vi "Tag Based Metadata Interface.vi"(0 "Save Path":path, 7 "Input Tags Path":path) -> ()   [LabVIEW 2020]
uses:
  <vilib>/Utility/miscctls.llb/LVPointTypeDef.ctl
  <vilib>/Utility/file.llb/Read Delimited Spreadsheet (string).vi
panel:
  in  "Clear All Tags":bool
  in  "Group Name Input":string
  in  "Clear Tags":bool
  in  "Remove Group":bool
  in  "Add Group":bool
  in  "Notes":string
  in  "Tag Group 6":bool
  in  "Tag Group 5":bool
  in  "Tag Group 4":bool
  in  "Tag Group 3":bool
  in  "Tag Group 2":bool
  in  "Tag Group 1":bool
  in  "Tag Group 0":bool
  in  "Metadata Tags":string[][](array[string])
  in  "Cancel":bool
  in  "Save":bool
  in  "Update Preset":bool
  in  "Save Preset":bool
  in  "Preset":u16(ring) items=["None", "Apple", "Bean", "My Test", "Test 01", "Test 02", "Test Two", "Zoo"]
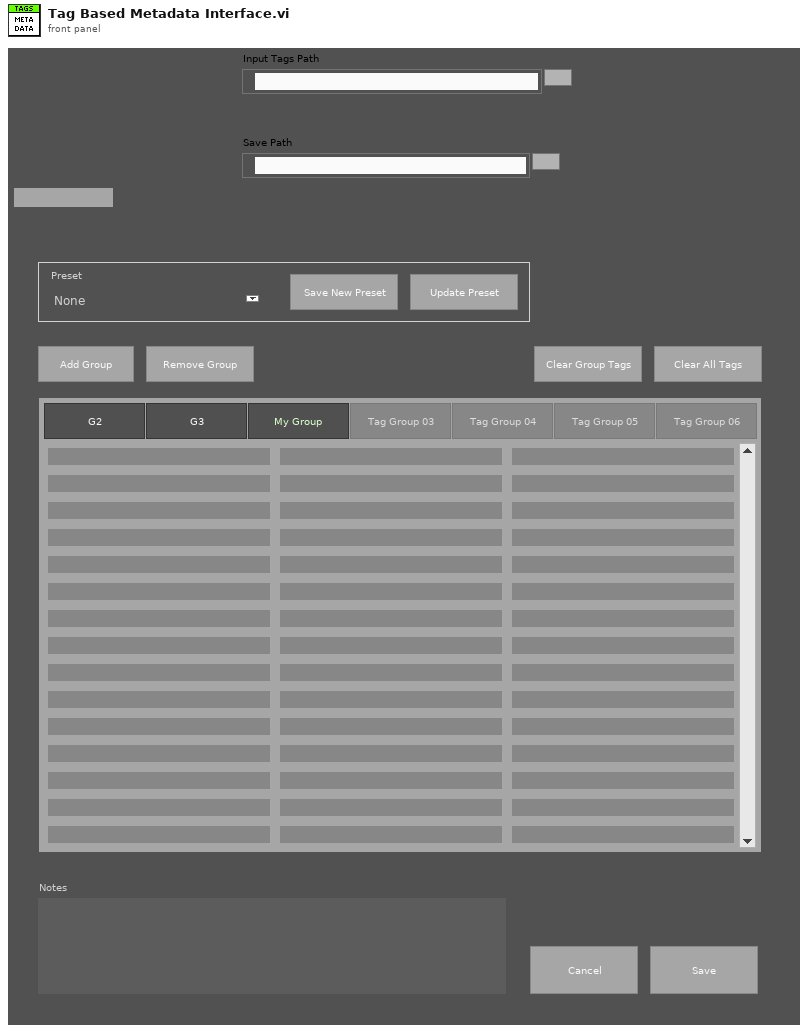
[diagram p1: front panel]
types:
  T1 = enum16{"Always On", "Always Off", "Off While Running"}
  T2 = typedef "LVPointTypeDef.ctl" = cluster{"Horizontal":i16, "Vertical":i16}
  T3 = enum8{"Enabled", "Disabled", "Disabled and Grayed Out"}
  T4 = typedef "LVRectTypeDef.ctl" = cluster{"Left":i16, "Top":i16, "Right":i16, "Bottom":i16}
  T5 = typedef "LVBoundsTypeDef.ctl" = cluster{"Width":u32, "Height":u32}
  T6 = enum32{"Invalid", "Standard", "Closed", "Hidden", "Minimized", "Maximized"}
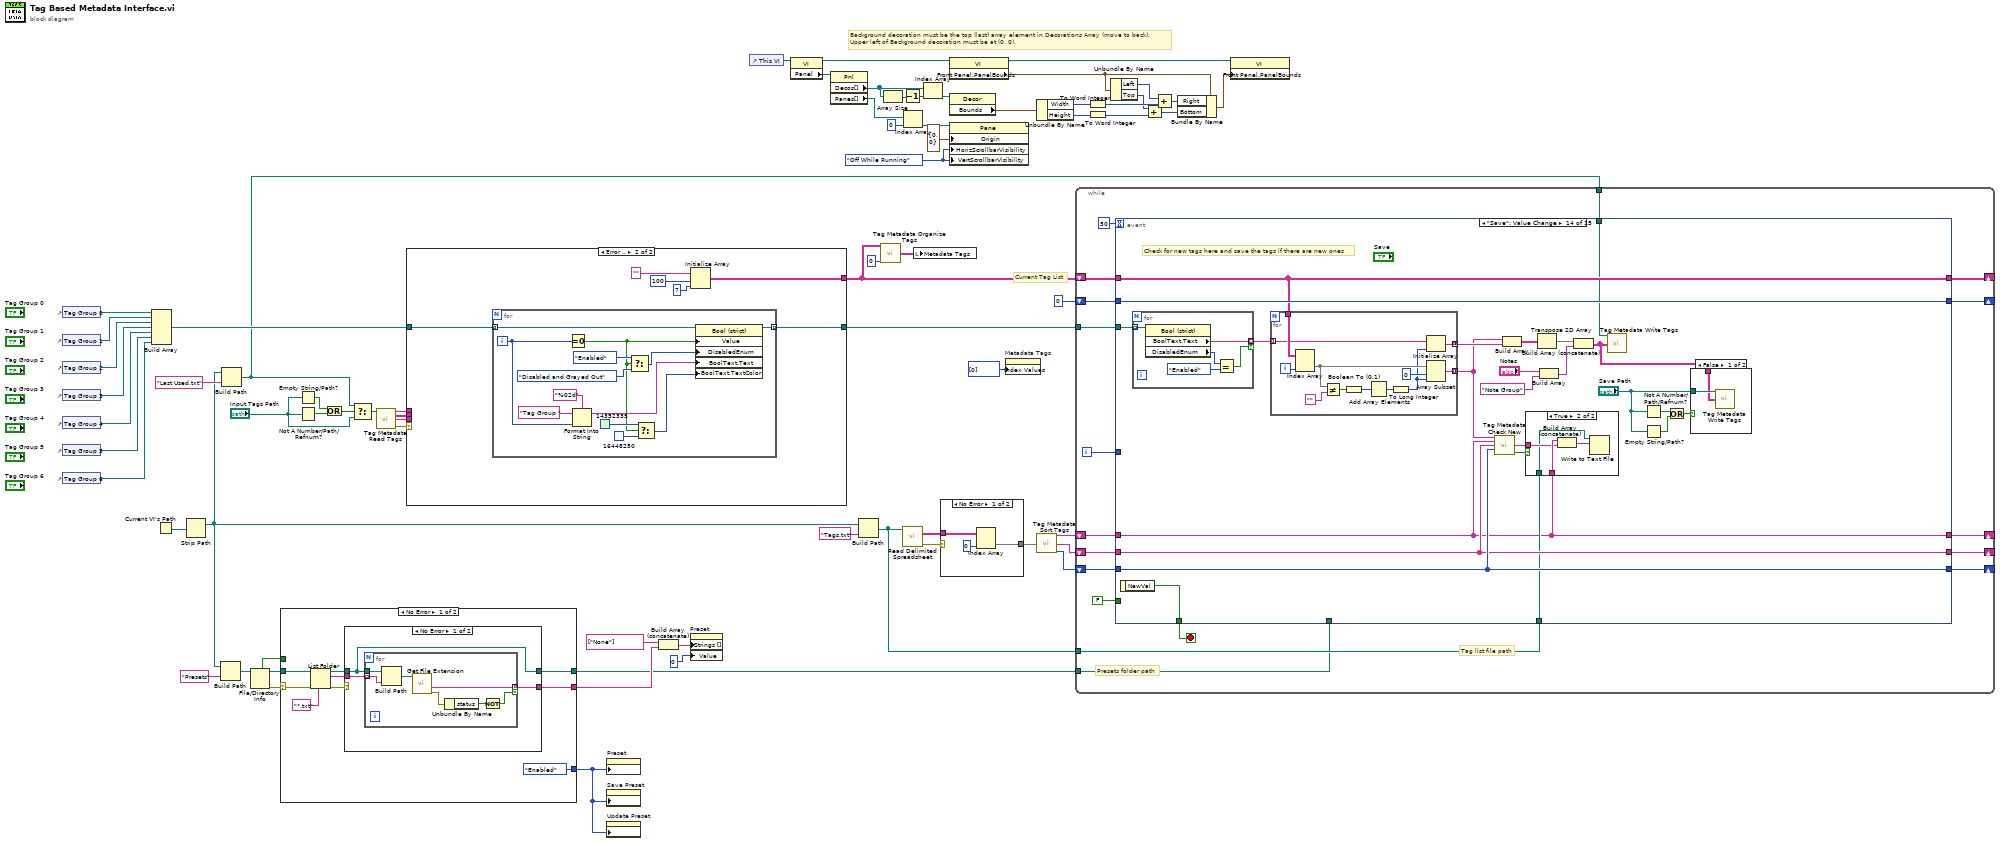
[diagram p0: block diagram]
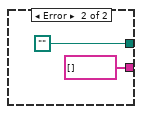
[diagram p2: hidden frame]
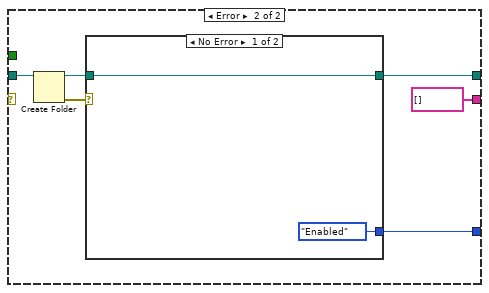
[diagram p3: hidden frame]
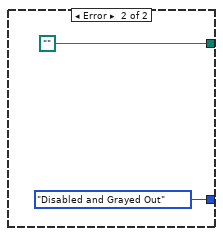
[diagram p4: hidden frame]
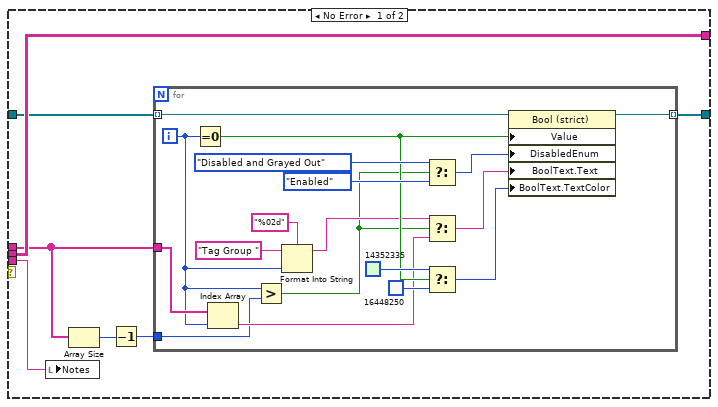
[diagram p5: hidden frame]
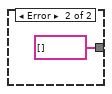
[diagram p6: hidden frame]
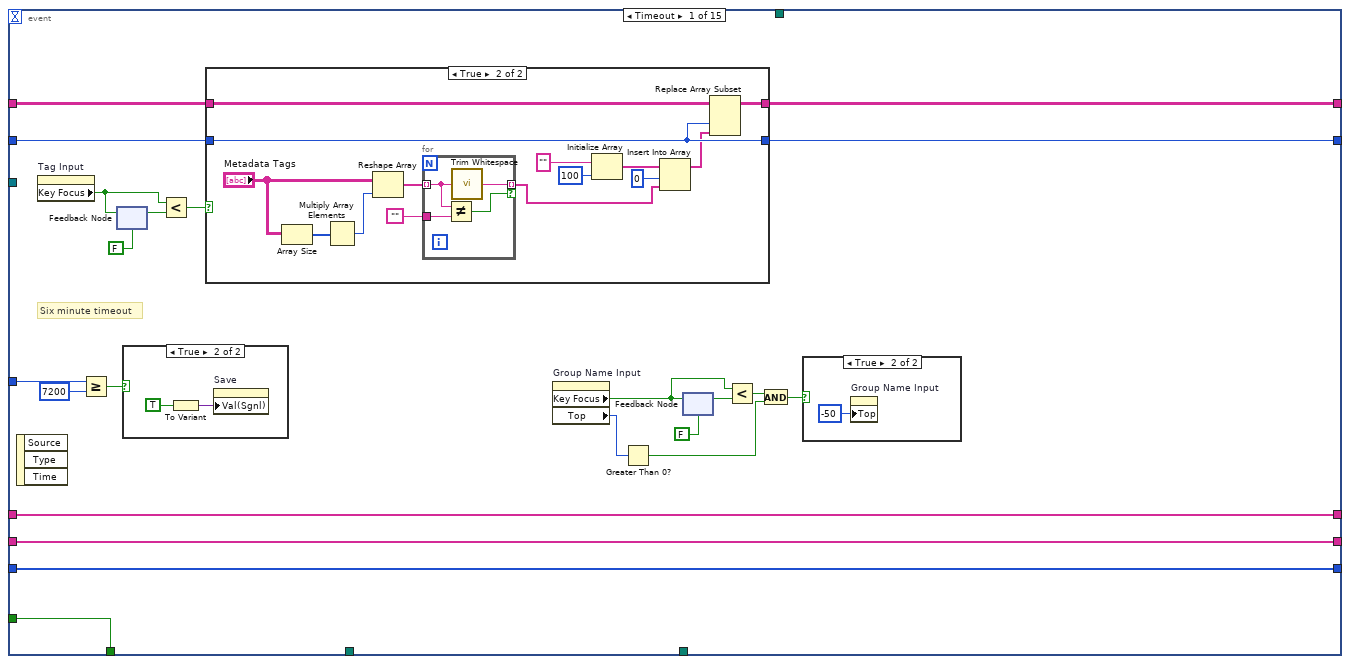
[diagram p7: hidden frame]
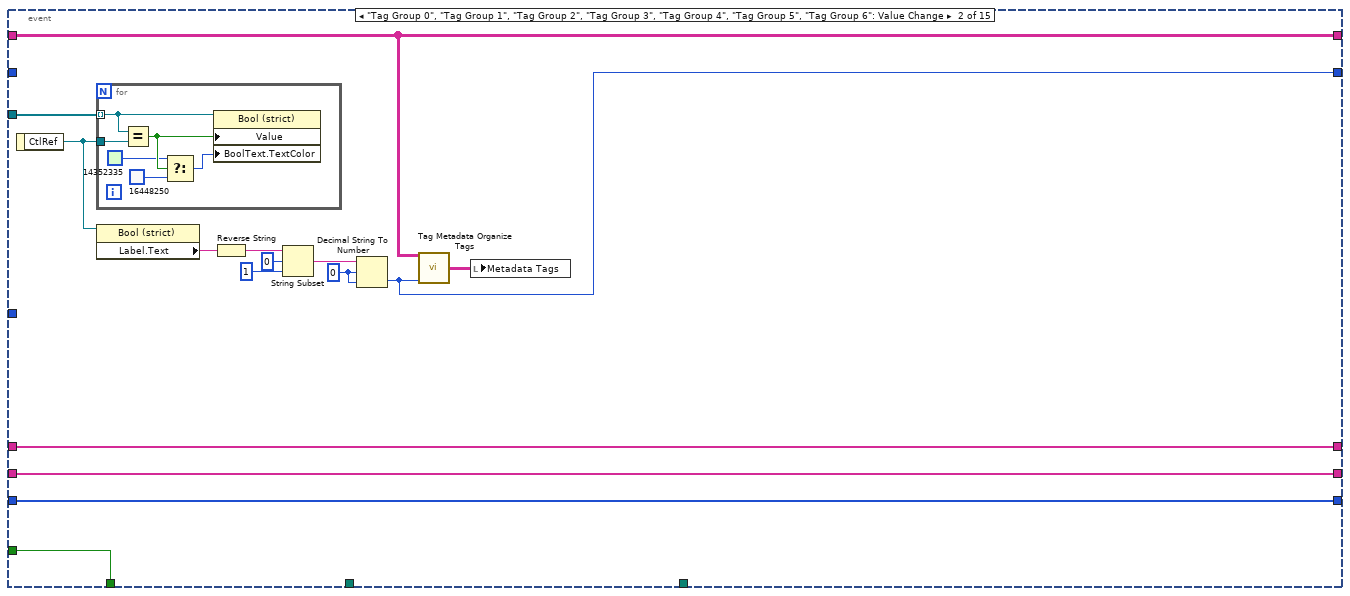
[diagram p11: hidden frame]
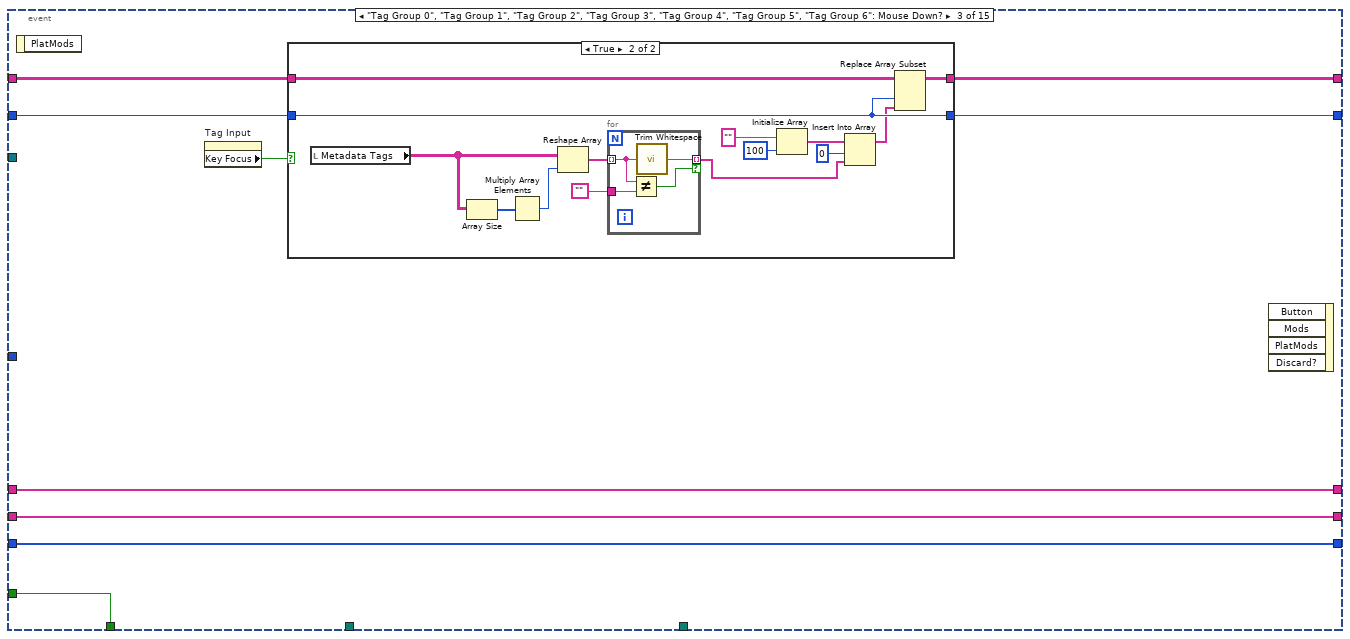
[diagram p12: hidden frame]
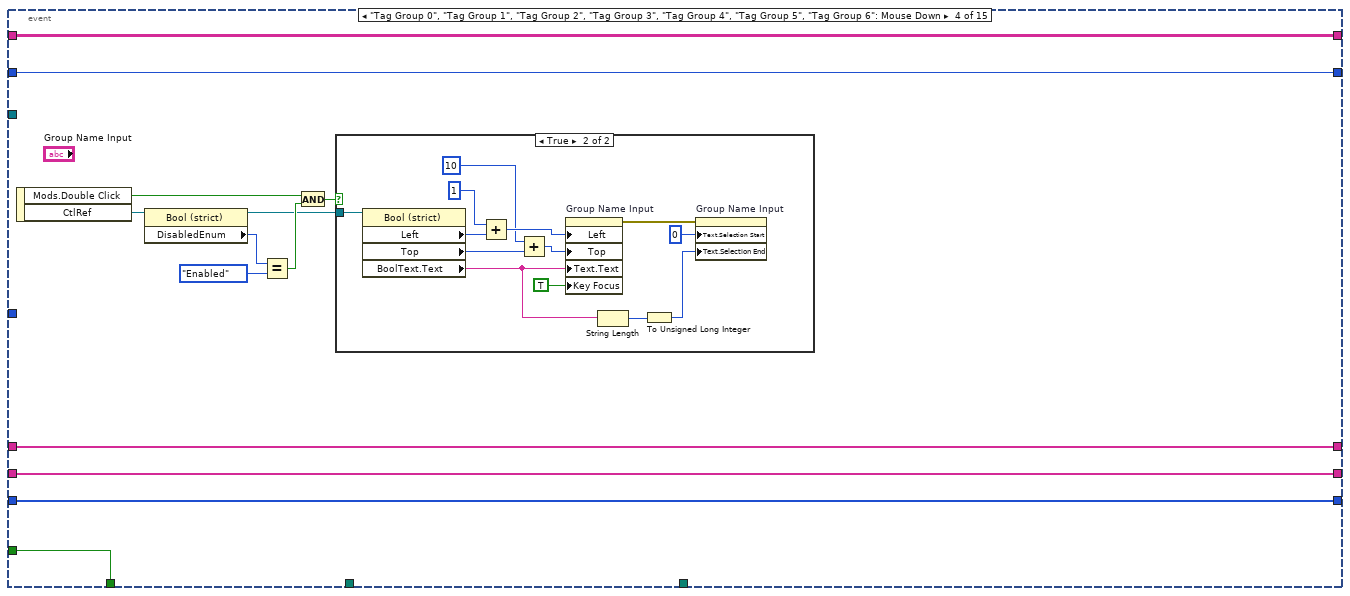
[diagram p14: hidden frame]
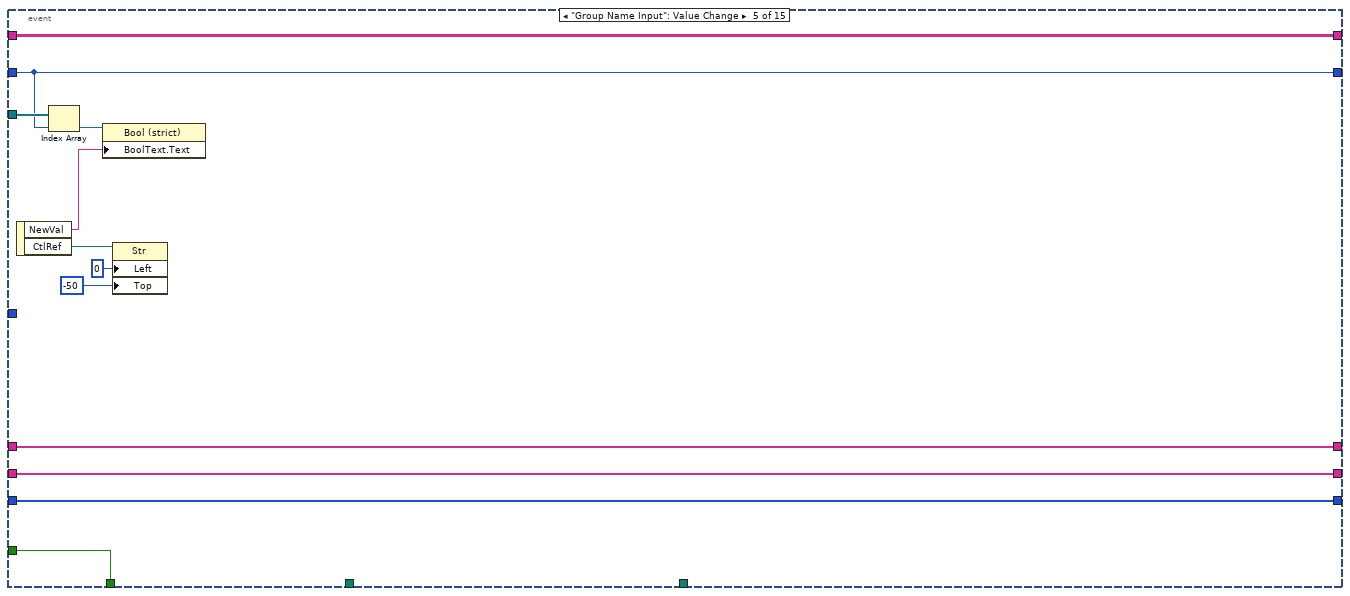
[diagram p16: hidden frame]
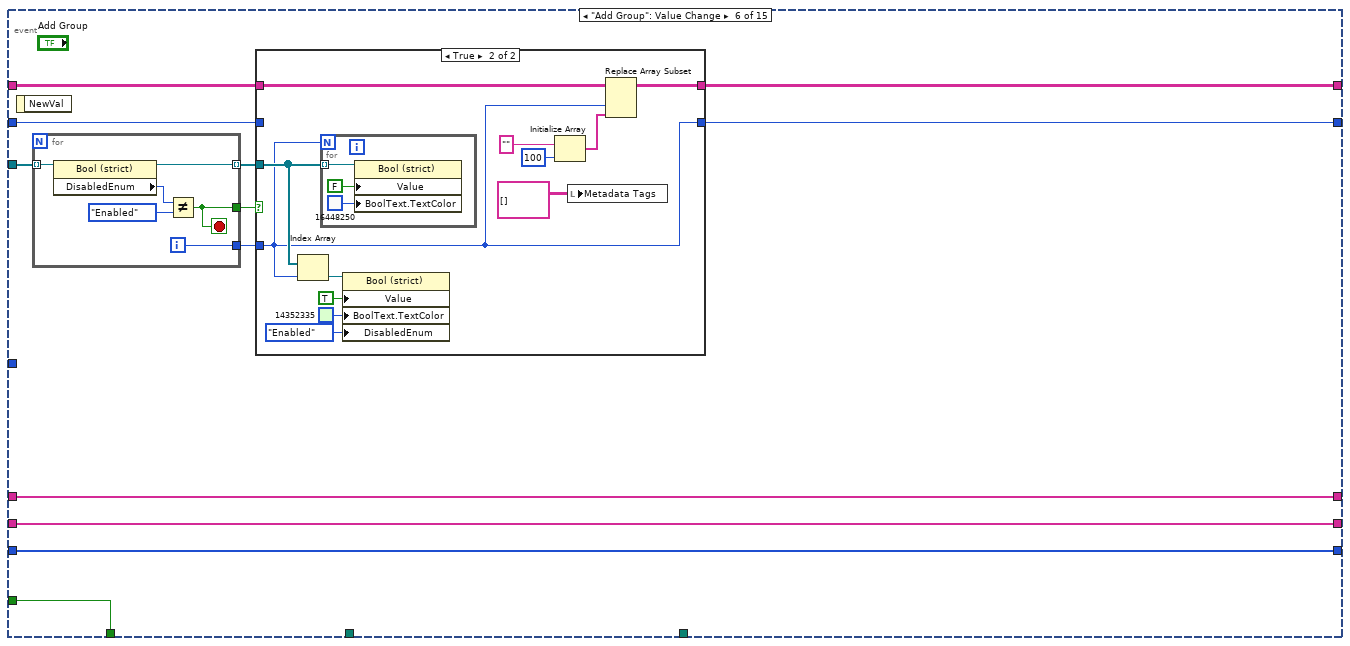
[diagram p17: hidden frame]
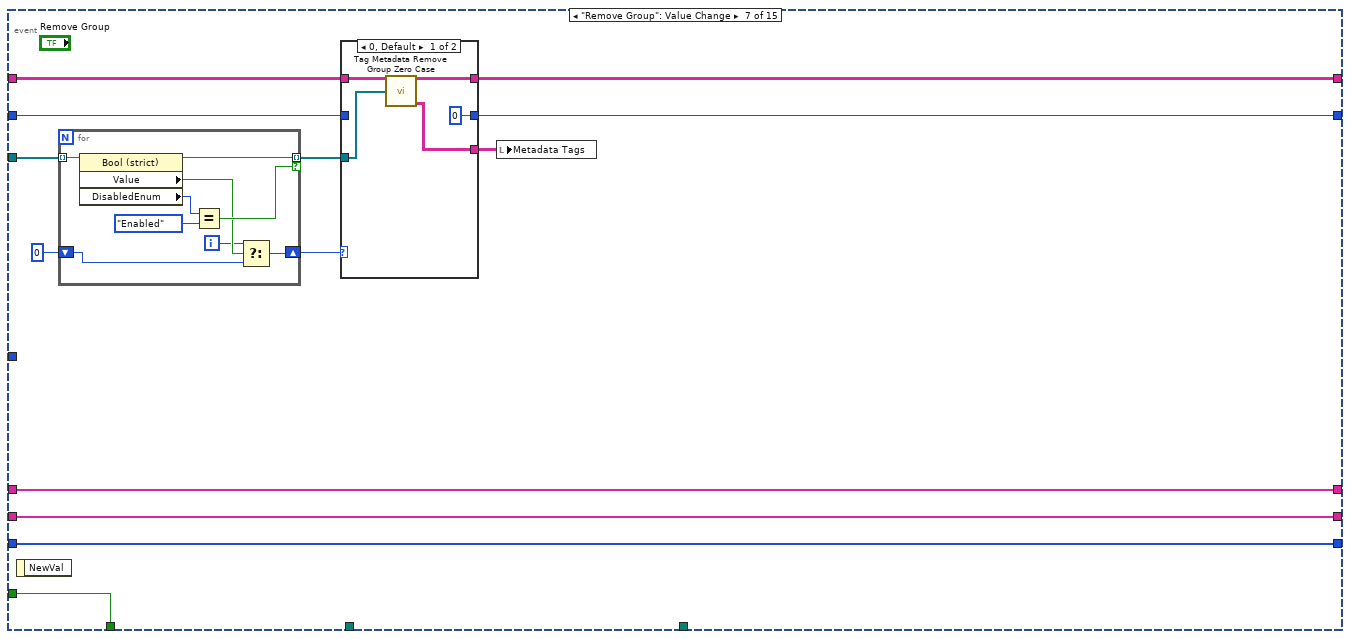
[diagram p19: hidden frame]
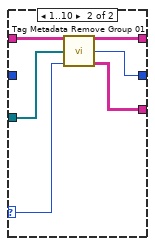
[diagram p20: hidden frame]
diagram:
  w61 = T1."Off While Running" ("Vertical Scrollbar Visibility")
  # "Current Tag List"
  # "Background decoration must be the top (last) array element in Decorations Array (move to back).\nUpper left of Background decoration must be at (0, 0)."
  n1 = control-ref of="Tag Group 0"() -> (w37:refnum<vi>)
  n2 = control-ref of="Tag Group 1"() -> (w36:refnum<vi>)
  n3 = control-ref of="Tag Group 2"() -> (w35:refnum<vi>)
  n4 = control-ref of="Tag Group 3"() -> (w34:refnum<vi>)
  n5 = control-ref of="Tag Group 4"() -> (w33:refnum<vi>)
  n6 = control-ref of="Tag Group 5"() -> (w32:refnum<vi>)
  n7 = control-ref of="Tag Group 6"() -> (w31:refnum<vi>)
  n8 = Build Array(w37, w36, w35, w34, w33, w32, w31) -> (w29:refnum<vi>[])
  n9 = Current VI's Path() -> (path=w44:path)
  n10 = Strip Path(path=w44) -> (stripped path=w6:path)  [unwired: 1 out]
  n11 = Build Path(base path=w6, name or relative path="Presets") -> (appended path=w20:path)
  n12 = Build Path(base path=w6, name or relative path="Last Used.txt") -> (appended path=w1:path)
  n13 = File/Directory Info(path=w20) -> (path out=w17:path, directory=w18:bool, error out=w19:errorcluster)  [unwired: 1 in, 4 out]
  n14 = case shown="No Error" w19 {
    selector: w19 -> [w78 _]
    tunnel: w18 -> [_ _]
    tunnel: w17 -> [w79 w97]
    tunnel: [w72 w94] -> w12
    tunnel: [w74 string[] []] -> w14
    tunnel: [T3."Enabled" ("Disabled") w92] -> w8
    frame No Error {
      n15 = List Folder(path=w79, pattern="*.txt", error in=w78) -> (path out=w75:path, filenames=w76:string[], error out=w73:errorcluster)  [unwired: 1 in, 1 out]
      n16 = case shown="No Error" w73 {
        tunnel: w76 -> [w82 _]
        tunnel: w75 -> [w80 _]
        tunnel: [w81 string[] []] -> w74
        tunnel: [w80 path ""] -> w72
        frame No Error {
          n17 = for {
            tunnel: w82 -> [w88] mode=indexing
            tunnel: w80 -> [w89]
            tunnel: [w86] -> w81 mode=indexing if=w83
            n18 = Build Path(base path=w89, name or relative path=w88) -> (appended path=w87:path)
            n19 = call <vilib>:"Get File Extension.vi"("file"=w87) -> ("error out"=w85:errorcluster, "filename without extension"=w86:string)  [unwired: 6 in, 3 out]
            n20 = Unbundle By Name(w85) -> ("status"=w84:bool)
            n21 = Not(x=w84) -> (.not. x?=w83:bool)
          }
        }
        frame Error {
        }
      }
    }
    frame Error {
      n22 = Create Folder(path (use dialog)=w97) -> (created path=w95:path, error out=w96:errorcluster)  [unwired: 2 in, 1 out]
      n23 = case shown="No Error" w96 {
        tunnel: w95 -> [w99 _]
        tunnel: [w99 path ""] -> w94
        tunnel: [T3."Enabled" ("Disabled") T3."Disabled and Grayed Out" ("Disabled")] -> w92
        frame No Error {
        }
        frame Error {
        }
      }
    }
  }
  n24 = Empty String/Path?(string/path="Input Tags Path") -> (empty?=w5:bool)
  n25 = Not A Number/Path/Refnum?(number/path/refnum="Input Tags Path") -> (NaN/Path/Refnum?=w4:bool)
  n26 = Or(x=w5, y=w4) -> (x .or. y?=w3:bool)
  n27 = Select(t=w1, s=w3, f="Input Tags Path") -> (s? t:f=w7:path)
  n28 = call "Tag Metadata Read Tags.vi"("Path"=w7) -> ("Group Names"=w24:string[], "Tags"=w23:string[][], "Notes"=w22:string, "Error Out"=w25:errorcluster)  [unwired: 11 in]
  n29 = case shown="Error .." w25 {
    tunnel: w29 -> [w107 w132]
    tunnel: [w106 w131] -> w28
    tunnel: [w108 w127] -> w11
    tunnel: w24 -> [w105 _]
    tunnel: w23 -> [w108 _]
    tunnel: w22 -> [w102 _]
    frame No Error {
      n30 = local write "Notes"(w102) -> ()
      n31 = Array Size(array=w105) -> (size(s)=w104:i32)
      n32 = Decrement(x=w104) -> (x-1=w103:i32)
      n33 = for {
        tunnel: w107 -> [w126] mode=indexing
        tunnel: [w125] -> w106 mode=indexing
        tunnel: w105 -> [w113]
        tunnel: w103 -> [w109]
        i -> [w111]
        n34 = Equal To 0?(x=w111) -> (x = 0?=w116:bool)
        n35 = Index Array(array=w113, index=w111) -> (element=w112:string)
        n36 = Greater?(x=w111, y=w109) -> (0:w110:bool)
        n37 = Format Into String(format string="%02d", initial string="Tag Group ", w111) -> (resulting string=w115:string)  [unwired: 1 in, 1 out]
        n38 = Select(t=T3."Disabled and Grayed Out" ("Disabled"), s=w110, f=T3."Enabled" ("Disabled")) -> (s? t:f=w123:T3)
        n39 = Select(t=w115, s=w110, f=w112) -> (s? t:f=w114:string)
        n40 = Select(t=u32 14352335 ("Color Box"), s=w116, f=u32 16448250) -> (s? t:f=w117:u32)
        n41 = property class="Bool (strict)"(reference=w126, "Value"=w116, "DisabledEnum"=w123, "BoolText.Text"=w114, "BoolText.TextColor"=w117) -> (reference out=w125:refnum<vi>)  [unwired: 1 in, 1 out]
      }
    }
    frame Error {
      n42 = for {
        tunnel: w132 -> [w145] mode=indexing
        tunnel: [w144] -> w131 mode=indexing
        i -> [w138]
        n43 = Equal To 0?(x=w138) -> (x = 0?=w133:bool)
        n44 = Format Into String(format string="%02d", initial string="Tag Group ", w138) -> (resulting string=w137:string)  [unwired: 1 in, 1 out]
        n45 = Select(t=T3."Enabled" ("Disabled"), s=w133, f=T3."Disabled and Grayed Out" ("Disabled")) -> (s? t:f=w142:T3)
        n46 = Select(t=u32 14352335 ("Color Box"), s=w133, f=u32 16448250) -> (s? t:f=w134:u32)
        n47 = property class="Bool (strict)"(reference=w145, "Value"=w133, "DisabledEnum"=w142, "BoolText.Text"=w137, "BoolText.TextColor"=w134) -> (reference out=w144:refnum<vi>)  [unwired: 1 in, 1 out]
      }
      n48 = Initialize Array("", 100 ("dimension size"), 7 ("dimension size")) -> (w127:string[][])
    }
  }
  n49 = property on="Preset" class="Ring (strict)"("DisabledEnum"=w8) -> ()  [unwired: 2 in, 2 out]
  n50 = property on="Save Preset" class="Bool"("DisabledEnum"=w8) -> ()  [unwired: 2 in, 2 out]
  n51 = property on="Update Preset" class="Bool"("DisabledEnum"=w8) -> ()  [unwired: 2 in, 2 out]
  n52 = Build Array (concatenate)(string[] ["None"] ("Strings []"), w14) -> (w15:string[])
  n53 = property on="Preset" class="Ring (strict)"("Strings []"=w15, "Value"=u16 0) -> ()  [unwired: 2 in, 2 out]
  n54 = control-ref of="This VI"() -> (w54:refnum<vi>)
  n55 = property class="VI"(reference=w54) -> (reference out=w62:refnum<vi>, "Panel"=w55:refnum<vi>)  [unwired: 1 in, 1 out]
  n56 = property class="Pnl"(reference=w55) -> ("Decos[]"=w39:refnum<vi>[], "Panes[]"=w58:refnum<vi>[])  [unwired: 1 in, 2 out]
  n57 = Build Path(base path=w6, name or relative path="Tags.txt") -> (appended path=w26:path)
  n58 = call "Tag Metadata Organize Tags.vi"("Current Tags"=w11, "Group Index"=0) -> ("Display Tags"=w9:string[][])  [unwired: 13 in]
  n59 = Array Size(array=w39) -> (size(s)=w53:i32)
  n60 = Decrement(x=w53) -> (x-1=w38:i32)
  n61 = call-poly <vilib>:"Read Delimited Spreadsheet.vi"("file path (dialog if empty)"=w26) -> ("all rows"=w42:string[][], "error out"=w41:errorcluster)  [unwired: 9 in, 4 out]
  n62 = Index Array(array=w58, index=0) -> (element=w57:refnum<vi>)
  n63 = local write "Metadata Tags"(w9) -> ()
  n64 = Index Array(array=w39, index=w38) -> (element=w60:refnum<vi>)
  n65 = case shown="No Error" w41 {
    tunnel: w42 -> [w148 _]
    tunnel: [w146 string[] [] ("all rows")] -> w40
    frame No Error {
      n66 = Index Array(array=w148, index (col)=0 ("disabled index (col)")) -> (element=w146:string[])  [unwired: 1 in]
    }
    frame Error {
    }
  }
  n67 = property class="VI"(reference=w62) -> (reference out=w64:refnum<vi>, "Front Panel.PanelBounds"=w65:T4)  [unwired: 1 in, 1 out]
  n68 = property class="Decor"(reference=w60) -> ("Bounds"=w63:T5)  [unwired: 1 in, 2 out]
  n69 = property class="Pane"(reference=w57, "Origin"=T2 {"Horizontal"=0, "Vertical"=0}, "HorizScrollbarVisibility"=w61, "VertScrollbarVisibility"=w61) -> ()  [unwired: 1 in, 2 out]
  n70 = property on="Metadata Tags" class="Arr (strict)"("Index Values"=u32[] [0]) -> ()  [unwired: 2 in, 2 out]
  n71 = Unbundle By Name(w63) -> ("Width"=w68:u32, "Height"=w70:u32)
  n72 = call "Tag Metadata Sort Tags.vi"("Tags"=w40) -> ("Sorted Tags"=w47:string[], "First Letters"=w46:string[], "Letter Indicies"=w45:i32[])  [unwired: 12 in]
  n73 = while {
    shift-right: [w160] -> _
    shift-left: w47 -> [w165]
    shift-right: [w161] -> _
    shift-left: w46 -> [w164]
    shift-right: [w162] -> _
    shift-left: w45 -> [w163]
    tunnel: w28 -> [w159]
    shift-right: [w152] -> _
    shift-left: w11 -> [w158]
    shift-right: [w156] -> _
    shift-left: 0 -> [w157]
    tunnel: w26 -> [w154]
    tunnel: w1 -> [w153]
    tunnel: w12 -> [w151]
    i -> [w150]
    stop <- w166 stop-if-true
    # "Presets folder path"
    # "Tag list file path"
    n74 = event shown="[13] \"Save\": Value Change" {
      selector: _ -> [_ _ _ _ _ _ _ _ _ _ _ _ _ _ _]
      dyn-events: _ -> [_ _ _ _ _ _ _ _ _ _ _ _ _ _ _]
      timeout: 50 -> [_ _ _ _ _ _ _ _ _ _ _ _ _ _ _]
      tunnel: FALSE -> [w189 w227 w242 w275 w300 w312 w348 w385 w409 w419 w441 w495 w536 _ _]
      tunnel: [w189 w227 w242 w275 w300 w312 w348 w385 w409 w419 w441 w495 w536 w597 TRUE ("NewVal")] -> w166
      tunnel: w165 -> [w188 w225 w241 w274 w299 w311 w347 w372 w408 w417 w440 w494 w535 w585 w623]
      tunnel: w164 -> [w187 w224 w240 w273 w298 w310 w346 w373 w407 w416 w439 w493 w534 w589 w622]
      tunnel: w163 -> [w186 w223 w239 w272 w297 w309 w345 w374 w406 w415 w438 w492 w533 w590 w621]
      tunnel: [w186 w223 w239 w272 w297 w309 w345 w374 w406 w415 w438 w492 w533 w590 w621] -> w162
      tunnel: [w187 w224 w240 w273 w298 w310 w346 w373 w407 w416 w439 w493 w534 w589 w622] -> w161
      tunnel: [w188 w225 w241 w274 w299 w311 w347 w372 w408 w417 w440 w494 w535 w585 w623] -> w160
      tunnel: w159 -> [_ w226 _ _ w292 w301 w344 _ _ _ w428 w482 w531 w595 _]
      tunnel: [w179 w214 w237 w271 w296 w303 w340 w370 w402 w410 w420 w481 w523 w593 w625] -> w152
      tunnel: w158 -> [w181 w214 w238 w271 w296 w304 w341 w370 w403 _ w423 w481 w530 w593 w625]
      tunnel: w157 -> [w180 _ w236 w270 w291 w307 w339 w371 w401 w414 w422 w491 w525 w596 w624]
      tunnel: [w178 w213 w235 w270 w291 w305 w338 w371 w401 w414 w421 w491 w524 w596 w624] -> w156
      tunnel: w154 -> [_ _ _ _ _ _ _ _ _ _ _ _ _ w586 _]
      tunnel: w153 -> [_ _ _ _ _ _ _ _ _ _ _ _ _ w579 _]
      tunnel: w151 -> [_ _ _ _ _ _ _ _ _ _ w430 w475 w528 _ _]
      tunnel: w150 -> [w170 _ _ _ _ _ _ _ _ _ _ _ _ _ _]
      event Timeout {
        # "Six minute timeout"
        n75 = event-data() -> ()  [unwired: 1 in, 3 out]
        n76 = property on="Tag Input" class="Str"() -> ("Key Focus"=w184:bool)  [unwired: 2 in, 2 out]
        n77 = Greater Or Equal?(x=w170, y=7200) -> (x >= y?=w168:bool)
        n78 = feedback-in #1(w184) -> ()
        n79 = feedback #1(FALSE ("Key Focus")) -> (w185:bool)
        n80 = case shown="True" w168 {
          frame False {
          }
          frame True {
            n81 = To Variant(anything=TRUE) -> (Variant=w190:variant)
            n82 = property on="Save" class="Bool"("Val(Sgnl)"=w190) -> ()  [unwired: 2 in, 2 out]
          }
        }
        n83 = Less?(x=w184, y=w185) -> (x < y?=w182:bool)
        n84 = case shown="True" w182 {
          tunnel: w181 -> [w194 w203]
          tunnel: w180 -> [w193 w201]
          tunnel: [w194 w202] -> w179
          tunnel: [w193 w201] -> w178
          frame False {
          }
          frame True {
            n85 = Array Size(array="Metadata Tags") -> (size(s)=w205:i32[])
            n86 = Multiply Array Elements(1:w205) -> (0:w207:i32)
            n87 = Reshape Array("Metadata Tags", w207) -> (w208:string[])
            n88 = for {
              tunnel: w208 -> [w211] mode=indexing
              tunnel: "" -> [w212]
              tunnel: [w210] -> w196 mode=indexing if=w209
              n89 = Not Equal?(x=w211, y=w212) -> (x != y?=w209:bool)
              n90 = call <vilib>:"Trim Whitespace.vi"("string"=w211) -> ("trimmed string"=w210:string)  [unwired: 1 in]
            }
            n91 = Initialize Array("", 100 ("dimension size")) -> (w200:string[])
            n92 = Insert Into Array(array=w200, index=0, new element=w196) -> (w195:string[])
            n93 = Replace Array Subset(array=w203, new element=w195, index (col)=w201) -> (w202:string[][])  [unwired: 1 in]
          }
        }
        n94 = property on="Group Name Input" class="Str"() -> ("Key Focus"=w175:bool, "Top"=w174:i32)  [unwired: 2 in, 2 out]
        n95 = Greater Than 0?(x=w174) -> (x > 0?=w172:bool)
        n96 = feedback #2(FALSE ("Key Focus")) -> (w177:bool)
        n97 = feedback-in #2(w175) -> ()
        n98 = Less?(x=w175, y=w177) -> (x < y?=w173:bool)
        n99 = And(x=w173, y=w172) -> (x .and. y?=w171:bool)
        n100 = case shown="True" w171 {
          frame False {
          }
          frame True {
            n101 = property on="Group Name Input" class="Str"("Top"=-50 ("Position:Top")) -> ()  [unwired: 2 in, 2 out]
          }
        }
      }
      event "Tag Group 0", "Tag Group 1", "Tag Group 2", "Tag Group 3", "Tag Group 4", "Tag Group 5", "Tag Group 6": Value Change {
        w216 = 0 ("offset")
        n102 = event-data() -> ("CtlRef"=w222:refnum<vi>)  [unwired: 1 in]
        n103 = for {
          tunnel: w226 -> [w232] mode=indexing
          tunnel: w222 -> [w233]
          n104 = Equal?(x=w232, y=w233) -> (x = y?=w231:bool)
          n105 = Select(t=u32 14352335 ("Color Box"), s=w231, f=u32 16448250) -> (s? t:f=w229:u32)
          n106 = property class="Bool (strict)"(reference=w232, "Value"=w231, "BoolText.TextColor"=w229) -> ()  [unwired: 1 in, 2 out]
        }
        n107 = property class="Bool (strict)"(reference=w222) -> ("Label.Text"=w221:string)  [unwired: 1 in, 2 out]
        n108 = Reverse String(1:w221) -> (0:w220:string)
        n109 = String Subset(string=w220, offset (0)=0, length (rest)=1 ("length (rest)")) -> (substring=w217:string)
        n110 = Decimal String To Number(string=w217, offset=w216, default (0L)=w216) -> (number=w213:i32)  [unwired: 1 out]
        n111 = call "Tag Metadata Organize Tags.vi"("Current Tags"=w214, "Group Index"=w213) -> ("Display Tags"=w215:string[][])  [unwired: 13 in]
        n112 = local write "Metadata Tags"(w215) -> ()
      }
      event "Tag Group 0", "Tag Group 1", "Tag Group 2", "Tag Group 3", "Tag Group 4", "Tag Group 5", "Tag Group 6": Mouse Down? {
        n113 = event-data() -> ()  [unwired: 1 in, 1 out]
        n114 = property on="Tag Input" class="Str"() -> ("Key Focus"=w234:bool)  [unwired: 2 in, 2 out]
        n115 = case shown="True" w234 {
          tunnel: w238 -> [w244 w254]
          tunnel: w236 -> [w243 w252]
          tunnel: [w244 w253] -> w237
          tunnel: [w243 w252] -> w235
          frame False {
          }
          frame True {
            n116 = local read "Metadata Tags"() -> (w245:string[][])
            n117 = Array Size(array=w245) -> (size(s)=w256:i32[])
            n118 = Multiply Array Elements(1:w256) -> (0:w257:i32)
            n119 = Reshape Array(w245, w257) -> (w258:string[])
            n120 = for {
              tunnel: w258 -> [w261] mode=indexing
              tunnel: "" -> [w262]
              tunnel: [w260] -> w247 mode=indexing if=w259
              n121 = Not Equal?(x=w261, y=w262) -> (x != y?=w259:bool)
              n122 = call <vilib>:"Trim Whitespace.vi"("string"=w261) -> ("trimmed string"=w260:string)  [unwired: 1 in]
            }
            n123 = Initialize Array("", 100 ("dimension size")) -> (w251:string[])
            n124 = Insert Into Array(array=w251, index=0, new element=w247) -> (w246:string[])
            n125 = Replace Array Subset(array=w254, new element=w246, index (col)=w252) -> (w253:string[][])  [unwired: 1 in]
          }
        }
        n126 = event-data() -> ()  [unwired: 5 in, 1 out]
      }
      event "Tag Group 0", "Tag Group 1", "Tag Group 2", "Tag Group 3", "Tag Group 4", "Tag Group 5", "Tag Group 6": Mouse Down {
        n127 = event-data() -> ("Mods.Double Click"=w266:bool, "CtlRef"=w269:refnum<vi>)  [unwired: 1 in]
        n128 = property class="Bool (strict)"(reference=w269) -> (reference out=w264:refnum<vi>, "DisabledEnum"=w268:T3)  [unwired: 1 in, 1 out]
        n129 = Equal?(x=w268, y=T3."Enabled") -> (x = y?=w265:bool)
        n130 = And(x=w266, y=w265) -> (x .and. y?=w263:bool)
        n131 = case shown="True" w263 {
          tunnel: w264 -> [_ w288]
          frame False {
          }
          frame True {
            n132 = property class="Bool (strict)"(reference=w288) -> ("Left"=w281:i32, "Top"=w278:i32, "BoolText.Text"=w285:string)  [unwired: 1 in, 2 out]
            n133 = Add(x=1 ("Left"), y=w281) -> (x+y=w279:i32)
            n134 = Add(x=10 ("Top"), y=w278) -> (x+y=w277:i32)
            n135 = property on="Group Name Input" class="Str"("Left"=w279, "Top"=w277, "Text.Text"=w285, "Key Focus"=TRUE) -> (error out=w287:errorcluster)  [unwired: 2 in, 1 out]
            n136 = String Length(string=w285) -> (length=w284:i32)
            n137 = To Unsigned Long Integer(number=w284) -> (unsigned 32bit integer=w283:u32)
            n138 = property on="Group Name Input" class="Str"(error in=w287, "Text.Selection Start"=u32 0 ("Text.Selection:Start"), "Text.Selection End"=w283) -> ()  [unwired: 1 in, 2 out]
          }
        }
      }
      event "Group Name Input": Value Change {
        n139 = event-data() -> ("NewVal"=w289:string, "CtlRef"=w295:refnum<vi>)  [unwired: 1 in]
        n140 = Index Array(array=w292, index=w291) -> (element=w290:refnum<vi>)
        n141 = property class="Bool (strict)"(reference=w290, "BoolText.Text"=w289) -> ()  [unwired: 1 in, 2 out]
        n142 = property class="Str"(reference=w295, "Left"=0 ("Position:Left"), "Top"=-50 ("Position:Top")) -> ()  [unwired: 1 in, 2 out]
      }
      event "Add Group": Value Change {
        n143 = event-data() -> ()  [unwired: 1 in, 1 out]
        n144 = for {
          tunnel: w301 -> [w334] mode=indexing
          tunnel: [w333] -> w302 mode=indexing
          tunnel: [w332] -> w308
          tunnel: [w331] -> w306
          i -> [w331]
          stop <- w332 stop-if-true
          n145 = property class="Bool (strict)"(reference=w334) -> (reference out=w333:refnum<vi>, "DisabledEnum"=w330:T3)  [unwired: 1 in, 1 out]
          n146 = Not Equal?(x=w330, y=T3."Enabled") -> (x != y?=w332:bool)
        }
        n147 = case shown="True" w308 {
          tunnel: w307 -> [w314 _]
          tunnel: w306 -> [_ w319]
          tunnel: [w314 w319] -> w305
          tunnel: w304 -> [w313 w322]
          tunnel: [w313 w321] -> w303
          tunnel: w302 -> [_ w320]
          frame False {
          }
          frame True {
            n148 = Index Array(array=w320, index=w319) -> (element=w318:refnum<vi>)
            n149 = for {
              N: w319 -> [_]
              tunnel: w320 -> [w327] mode=indexing
              n150 = property class="Bool (strict)"(reference=w327, "Value"=FALSE, "BoolText.TextColor"=u32 16448250) -> ()  [unwired: 1 in, 2 out]
            }
            n151 = property class="Bool (strict)"(reference=w318, "Value"=TRUE, "BoolText.TextColor"=u32 14352335 ("Color Box"), "DisabledEnum"=T3."Enabled" ("Disabled")) -> ()  [unwired: 1 in, 2 out]
            n152 = Initialize Array("", 100 ("dimension size")) -> (w324:string[])
            n153 = local write "Metadata Tags"(string[][] []) -> ()
            n154 = Replace Array Subset(array=w322, new element=w324, index (col)=w319) -> (w321:string[][])  [unwired: 1 in]
          }
        }
      }
      event "Remove Group": Value Change {
        n155 = event-data() -> ()  [unwired: 1 in, 1 out]
        n156 = for {
          tunnel: w344 -> [w368] mode=indexing
          tunnel: [w365] -> w342 mode=indexing if=w364
          shift-right: [w361] -> w337
          shift-left: 0 -> [w362]
          i -> [w360]
          n157 = property class="Bool (strict)"(reference=w368) -> (reference out=w365:refnum<vi>, "Value"=w363:bool, "DisabledEnum"=w367:T3)  [unwired: 1 in, 1 out]
          n158 = Equal?(x=w367, y=T3."Enabled") -> (x = y?=w364:bool)
          n159 = Select(t=w360, s=w363, f=w362) -> (s? t:f=w361:i32)
        }
        n160 = case shown="0, Default" w337 {
          selector: w337 -> [_ w358]
          tunnel: w342 -> [w350 w357]
          tunnel: w341 -> [w353 w359]
          tunnel: [w352 w355] -> w340
          tunnel: w339 -> [_ _]
          tunnel: [0 ("Update Index") w356] -> w338
          tunnel: [w351 w354] -> w336
          frame 0, Default {
            n161 = call "Tag Metadata Remove Group Zero Case.vi"("Tags Array"=w353, "Boolean Refs Array"=w350) -> ("Updated Tag Array"=w352:string[][], "Current Tags"=w351:string[][])  [unwired: 12 in]
          }
          frame 1..10 {
            n162 = call "Tag Metadata Remove Group 01.vi"("Tags Array"=w359, "Boolean Refs Array"=w357, "Group Index"=w358) -> ("Updated Tag Array"=w355:string[][], "Update Index"=w356:i32, "Current Tags"=w354:string[][])  [unwired: 10 in]
          }
        }
        n163 = local write "Metadata Tags"(w336) -> ()
      }
      event "Metadata Tags": Value Change {
        w379 = refnum<vi> refnum  # String
        n164 = event-data() -> ("CtlRef"=w383:refnum<vi>)  [unwired: 1 in]
        n165 = property class="Arr (strict)" props=["Array Element", "Array Element", "Value", "Key Focus"](reference=w383) -> ("Array Element"=w380:refnum<vi>, "Array Element.Value"=w376:variant)  [unwired: 1 in, 3 out]
        n166 = Variant To Data(type="", Variant=w376) -> (data=w378:string)  [unwired: 1 in, 1 out]
        n167 = To More Specific Class(target class=w379, reference=w380) -> (specific class reference=w369:refnum<vi>)  [unwired: 1 in, 1 out]
        n168 = call "Popup Menu Get State.vi"() -> ("FP State"=w382:T6, "Error Out"=w381:errorcluster)  [unwired: 14 in]
        n169 = call "Tag Metadata AutoComplete Items.vi"("Input String"=w378, "Match Limit"=10, "Sorted Tags"=w372, "First Letters"=w373, "Letter Indicies"=w374) -> ("AutoComplete"=w375:string[])  [unwired: 10 in]
        n170 = case shown="\"Standard\"" w382 {
          tunnel: w369 -> [_ w391 _]
          tunnel: w381 -> [_ w387 w395]
          tunnel: w375 -> [_ w386 w392]
          frame Default {
          }
          frame "Closed" {
            n171 = control-ref of="This VI"() -> (w390:refnum<vi>)
            n172 = call "Popup Menu Get XY.vi"("VI Ref"=w390, "Str Ctrl Ref"=w391, "Errror In"=w387) -> ("Screen Coordinates"=w389:T2, "Error Out"=w388:errorcluster)  [unwired: 11 in]
            n173 = call "Popup Menu Start.vi"("VI Ref"=w390, "Str Ctrl Ref"=w391, "Initial Menu Options"=w386, "Error In"=w388, "XY Position"=w389) -> ()  [unwired: 10 in, 1 out]
          }
          frame "Standard" {
            n174 = Array Size(array=w392) -> (size(s)=w394:i32)
            n175 = Greater Than 0?(x=w394) -> (x > 0?=w393:bool)
            n176 = case shown="False" w393 {
              tunnel: w395 -> [w396 w398]
              tunnel: w392 -> [_ w397]
              frame False {
                n177 = call "Popup Menu Close.vi"("Error In"=w396) -> ()  [unwired: 14 in, 1 out]
              }
              frame True {
                n178 = call "Popup Menu Update Items.vi"("Menu Items"=w397, "Error In"=w398) -> ()  [unwired: 13 in, 1 out]
              }
            }
          }
        }
      }
      event "Clear Tags": Value Change {
        n179 = event-data() -> ()  [unwired: 1 in, 6 out]
        n180 = Initialize Array("", 100 ("dimension size")) -> (w400:string[])
        n181 = local write "Metadata Tags"(string[][] []) -> ()
        n182 = Replace Array Subset(array=w403, new element=w400, index (col)=w401) -> (w402:string[][])  [unwired: 1 in]
      }
      event "Clear All Tags": Value Change {
        n183 = event-data() -> ()  [unwired: 1 in, 6 out]
        n184 = local write "Metadata Tags"(string[][] []) -> ()
        n185 = Initialize Array("", 100 ("dimension size"), 7 ("dimension size")) -> (w410:string[][])
      }
      event "Preset": Value Change {
        n186 = event-data() -> ("CtlRef"=w437:refnum<vi>, "NewVal"=w435:u16)  [unwired: 1 in]
        n187 = property class="Ring (strict)"(reference=w437) -> ("Strings []"=w436:string[])  [unwired: 1 in, 2 out]
        n188 = To Long Integer(number=w435) -> (32bit integer=w434:i32)
        n189 = Index Array(array=w436, index=w434) -> (element=w433:string)
        n190 = Concatenate Strings(w433, ".txt" ("string")) -> (w431:string)
        n191 = Build Path(base path=w430, name or relative path=w431) -> (appended path=w429:path)
        n192 = call "Tag Metadata Read Tags.vi"("Path"=w429) -> ("Group Names"=w427:string[], "Tags"=w426:string[][], "Notes"=w425:string, "Error Out"=w424:errorcluster)  [unwired: 11 in]
        n193 = case shown="No Error" w424 {
          tunnel: w428 -> [w450 _]
          tunnel: [w442 w469] -> w420
          tunnel: w427 -> [w449 _]
          tunnel: w426 -> [w442 _]
          tunnel: w425 -> [w446 _]
          tunnel: w423 -> [_ w469]
          tunnel: w422 -> [_ w468]
          tunnel: [0 w468] -> w421
          frame No Error {
            n194 = local write "Notes"(w446) -> ()
            n195 = Array Size(array=w449) -> (size(s)=w448:i32)
            n196 = call "Tag Metadata Organize Tags.vi"("Current Tags"=w442, "Group Index"=0) -> ("Display Tags"=w444:string[][])  [unwired: 13 in]
            n197 = Decrement(x=w448) -> (x-1=w447:i32)
            n198 = local write "Metadata Tags"(w444) -> ()
            n199 = for {
              tunnel: w450 -> [w467] mode=indexing
              tunnel: w449 -> [w455]
              tunnel: w447 -> [w451]
              i -> [w453]
              n200 = Equal To 0?(x=w453) -> (x = 0?=w458:bool)
              n201 = Index Array(array=w455, index=w453) -> (element=w454:string)
              n202 = Greater?(x=w453, y=w451) -> (0:w452:bool)
              n203 = Format Into String(format string="%02d", initial string="Tag Group ", w453) -> (resulting string=w457:string)  [unwired: 1 in, 1 out]
              n204 = Select(t=T3."Disabled and Grayed Out" ("Disabled"), s=w452, f=T3."Enabled" ("Disabled")) -> (s? t:f=w465:T3)
              n205 = Select(t=w457, s=w452, f=w454) -> (s? t:f=w456:string)
              n206 = Select(t=u32 14352335 ("Color Box"), s=w458, f=u32 16448250) -> (s? t:f=w459:u32)
              n207 = property class="Bool (strict)"(reference=w467, "Value"=w458, "DisabledEnum"=w465, "BoolText.Text"=w456, "BoolText.TextColor"=w459) -> ()  [unwired: 1 in, 2 out]
            }
          }
          frame Error {
          }
        }
      }
      event "Save Preset": Value Change {
        n208 = event-data() -> ()  [unwired: 1 in, 6 out]
        n209 = for {
          tunnel: w482 -> [w520] mode=indexing
          tunnel: [w518] -> w490 mode=indexing if=w517
          n210 = property class="Bool (strict)"(reference=w520) -> ("BoolText.Text"=w518:string, "DisabledEnum"=w519:T3)  [unwired: 1 in, 2 out]
          n211 = Equal?(x=w519, y=T3."Enabled") -> (x = y?=w517:bool)
        }
        n212 = call "Tag Metadata Get User Input.vi"("Dialog Message"="Preset Name") -> ("User Input"=w472:string, "Canceled?"=w474:bool)  [unwired: 13 in]
        n213 = for {
          tunnel: w490 -> [w508] mode=indexing
          tunnel: w481 -> [w516]
          tunnel: [w506] -> w488 mode=concatenating
          tunnel: [w505] -> w489 mode=concatenating
          i -> [w515]
          n214 = Index Array(array=w516, index (col)=w515) -> (element=w511:string[])  [unwired: 1 in]
          n215 = Not Equal?(x=w511, y="") -> (x != y?=w513:bool[])
          n216 = Boolean To (0,1)(Boolean=w513) -> (0, 1=w512:i16[])
          n217 = Add Array Elements(numeric array=w512) -> (sum=w510:i16)
          n218 = To Long Integer(number=w510) -> (32bit integer=w507:i32)
          n219 = Initialize Array(w508, w507) -> (w505:string[])
          n220 = Array Subset(array=w511, index=0, length=w507) -> (w506:string[])
        }
        n221 = Concatenate Strings(w472, ".txt" ("string")) -> (w476:string)
        n222 = Build Path(base path=w475, name or relative path=w476) -> (appended path=w473:path)
        n223 = local read "Notes"() -> (w480:string)
        n224 = control-ref of="Preset"() -> (w479:refnum<vi>)
        n225 = Build Array(w488, w489) -> (w485:string[][])
        n226 = property class="Ring (strict)"(reference=w479) -> (reference out=w470:refnum<vi>, "Strings []"=w471:string[])  [unwired: 1 in, 1 out]
        n227 = Transpose 2D Array(2D array=w485) -> (transposed array=w484:string[][])
        n228 = Build Array(w480, "Note Group" ("string")) -> (w486:string[])
        n229 = Build Array (concatenate)(w484, w486) -> (w483:string[][])
        n230 = case shown="True" w474 {
          tunnel: w483 -> [w504 _]
          tunnel: w473 -> [w503 _]
          tunnel: w472 -> [w501 _]
          tunnel: w471 -> [w502 _]
          tunnel: w470 -> [w499 _]
          frame False {
            n231 = call "Tag Metadata Write Tags.vi"("File Path"=w503, "Tags Group Array"=w504) -> ()  [unwired: 13 in, 1 out]
            n232 = Build Array (concatenate)(w502, w501) -> (w496:string[])
            n233 = Array Size(array=w496) -> (size(s)=w500:i32)
            n234 = Decrement(x=w500) -> (x-1=w498:i32)
            n235 = To Unsigned Word Integer(number=w498) -> (unsigned 16bit integer=w497:u16)
            n236 = property class="Ring (strict)"(reference=w499, "Strings []"=w496, "Value"=w497) -> ()  [unwired: 1 in, 2 out]
          }
          frame True {
          }
        }
      }
      event "Update Preset": Value Change {
        n237 = event-data() -> ()  [unwired: 1 in, 6 out]
        n238 = control-ref of="Preset"() -> (w529:refnum<vi>)
        n239 = for {
          tunnel: w531 -> [w572] mode=indexing
          tunnel: [w570] -> w532 mode=indexing if=w569
          n240 = property class="Bool (strict)"(reference=w572) -> ("BoolText.Text"=w570:string, "DisabledEnum"=w571:T3)  [unwired: 1 in, 2 out]
          n241 = Equal?(x=w571, y=T3."Enabled") -> (x = y?=w569:bool)
        }
        n242 = property class="Ring (strict)"(reference=w529) -> ("Strings []"=w527:string[], "Value"=w526:u16)  [unwired: 1 in, 2 out]
        n243 = To Long Integer(number=w526) -> (32bit integer=w522:i32)
        n244 = case shown="Default" w522 {
          selector: w522 -> [_ w539]
          tunnel: w532 -> [_ w556]
          tunnel: w530 -> [w538 w540]
          tunnel: w528 -> [_ w545]
          tunnel: w527 -> [_ w543]
          tunnel: w525 -> [w537 w541]
          tunnel: [w537 w541] -> w524
          tunnel: [w538 w540] -> w523
          frame 0 {
          }
          frame Default {
            n245 = Index Array(array=w543, index=w539) -> (element=w542:string)
            n246 = for {
              tunnel: w556 -> [w560] mode=indexing
              tunnel: w540 -> [w568]
              tunnel: [w558] -> w554 mode=concatenating
              tunnel: [w557] -> w555 mode=concatenating
              i -> [w567]
              n247 = Index Array(array=w568, index (col)=w567) -> (element=w563:string[])  [unwired: 1 in]
              n248 = Not Equal?(x=w563, y="") -> (x != y?=w565:bool[])
              n249 = Boolean To (0,1)(Boolean=w565) -> (0, 1=w564:i16[])
              n250 = Add Array Elements(numeric array=w564) -> (sum=w562:i16)
              n251 = To Long Integer(number=w562) -> (32bit integer=w559:i32)
              n252 = Initialize Array(w560, w559) -> (w557:string[])
              n253 = Array Subset(array=w563, index=0, length=w559) -> (w558:string[])
            }
            n254 = Concatenate Strings(w542, ".txt" ("string")) -> (w546:string)
            n255 = Build Path(base path=w545, name or relative path=w546) -> (appended path=w544:path)
            n256 = local read "Notes"() -> (w548:string)
            n257 = Build Array(w554, w555) -> (w551:string[][])
            n258 = Transpose 2D Array(2D array=w551) -> (transposed array=w550:string[][])
            n259 = Build Array(w548, "Note Group" ("string")) -> (w552:string[])
            n260 = Build Array (concatenate)(w550, w552) -> (w549:string[][])
            n261 = call "Tag Metadata Write Tags.vi"("File Path"=w544, "Tags Group Array"=w549) -> ()  [unwired: 13 in, 1 out]
          }
        }
      }
      event "Save": Value Change {
        # "Check for new tags here and save the tags if there are new ones"
        n262 = event-data() -> ("NewVal"=w597:bool)  [unwired: 1 in]
        n263 = for {
          tunnel: w595 -> [w619] mode=indexing
          tunnel: [w617] -> w594 mode=indexing if=w616
          n264 = property class="Bool (strict)"(reference=w619) -> ("BoolText.Text"=w617:string, "DisabledEnum"=w618:T3)  [unwired: 1 in, 2 out]
          n265 = Equal?(x=w618, y=T3."Enabled") -> (x = y?=w616:bool)
        }
        n266 = for {
          tunnel: w594 -> [w607] mode=indexing
          tunnel: w593 -> [w615]
          tunnel: [w605] -> w591 mode=concatenating
          tunnel: [w604] -> w592 mode=concatenating
          i -> [w614]
          n267 = Index Array(array=w615, index (col)=w614) -> (element=w610:string[])  [unwired: 1 in]
          n268 = Not Equal?(x=w610, y="") -> (x != y?=w612:bool[])
          n269 = Boolean To (0,1)(Boolean=w612) -> (0, 1=w611:i16[])
          n270 = Add Array Elements(numeric array=w611) -> (sum=w609:i16)
          n271 = To Long Integer(number=w609) -> (32bit integer=w606:i32)
          n272 = Initialize Array(w607, w606) -> (w604:string[])
          n273 = Array Subset(array=w610, index=0, length=w606) -> (w605:string[])
        }
        n274 = call "Tag Metadata Check New.vi"("Tags"=w591, "Sorted Tags"=w585, "First Letters"=w589, "Letter Indicies"=w590) -> ("New Tags"=w587:string[], "New Tags Bool"=w588:bool)  [unwired: 10 in]
        n275 = Build Array(w591, w592) -> (w581:string[][])
        n276 = case shown="True" w588 {
          tunnel: w587 -> [_ w602]
          tunnel: w586 -> [_ w600]
          tunnel: w585 -> [_ w603]
          frame False {
          }
          frame True {
            n277 = Build Array (concatenate)(w603, w602) -> (w601:string[])
            n278 = Write to Text File(file (use dialog)=w600, text=w601) -> ()  [unwired: 2 in, 3 out]
          }
        }
        n279 = Transpose 2D Array(2D array=w581) -> (transposed array=w580:string[][])
        n280 = Build Array("Notes", "Note Group" ("string")) -> (w582:string[])
        n281 = Build Array (concatenate)(w580, w582) -> (w574:string[][])
        n282 = call "Tag Metadata Write Tags.vi"("File Path"=w579, "Tags Group Array"=w574) -> ()  [unwired: 13 in, 1 out]
        n283 = Not A Number/Path/Refnum?(number/path/refnum="Save Path") -> (NaN/Path/Refnum?=w578:bool)
        n284 = Empty String/Path?(string/path="Save Path") -> (empty?=w577:bool)
        n285 = Or(x=w578, y=w577) -> (x .or. y?=w576:bool)
        n286 = case shown="False" w576 {
          tunnel: "Save Path" -> [w599 _]
          tunnel: w574 -> [w598 _]
          frame False {
            n287 = call "Tag Metadata Write Tags.vi"("File Path"=w599, "Tags Group Array"=w598) -> ()  [unwired: 13 in, 1 out]
          }
          frame True {
          }
        }
      }
      event "Cancel": Value Change {
        n288 = event-data() -> ()  [unwired: 1 in, 3 out]
      }
    }
  }
  n289 = To Word Integer(number=w68) -> (16bit integer=w69:i16)
  n290 = To Word Integer(number=w70) -> (16bit integer=w49:i16)
  n291 = Unbundle By Name(w65) -> ("Left"=w67:i16, "Top"=w51:i16)
  n292 = Add(x=w51, y=w49) -> (x+y=w50:i16)
  n293 = Add(x=w67, y=w69) -> (x+y=w52:i16)
  n294 = Bundle By Name(cluster=w65, "Right"=w52, "Bottom"=w50) -> (w66:T4)
  n295 = property class="VI"(reference=w64, "Front Panel.PanelBounds"=w66) -> ()  [unwired: 1 in, 2 out]
